vi "MainSimulator_edit.vi"(6 "L2":dbl=130.0, 7 "L1":dbl=100.0, 8 "origin":cluster{"X":dbl, "Y":dbl}={"X"=200.0, "Y"=250.0}, 9 "a":dbl=20.0, 10 "beta 2":dbl(slide)=43.24022346368716 scale=-180.0..180.0, 11 "beta 1":dbl(slide)=43.24022346368716 scale=-180.0..180.0) -> (1 "3D Picture":refnum<vi>(3d-picture), 3 "Canvas":picture)   [LabVIEW 2020]
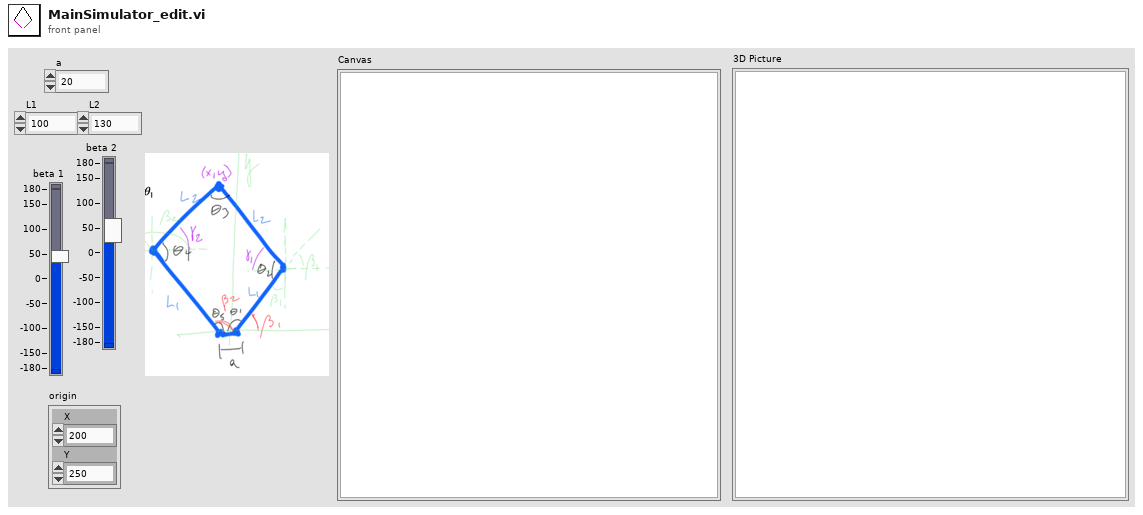
[diagram p1: front panel]
types:
  T1 = cluster{"Color":u32, "Length":dbl, "Base position":cluster{"X":dbl, "Y":dbl}, "Joint Angle":dbl}
  T2 = cluster{"Color":u32, "Length":dbl, "Base position":cluster{"X":dbl, "Y":dbl}, "Joint Angle":dbl}[]
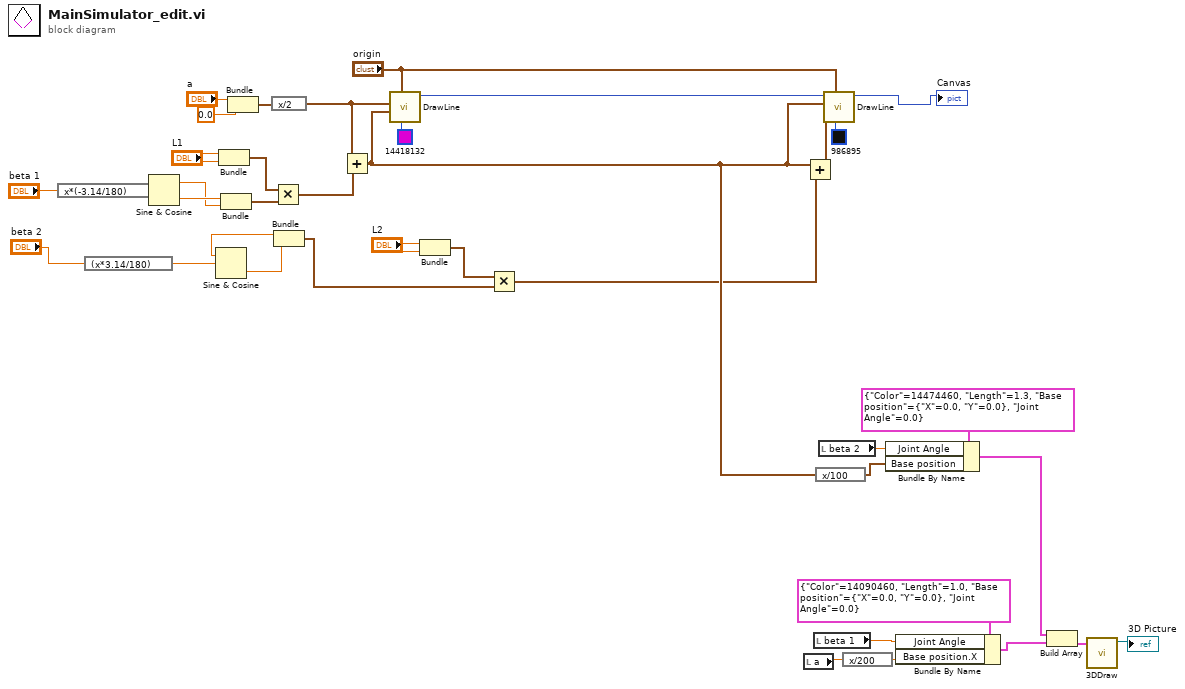
[diagram p0: block diagram]
diagram:
  n1 = expression code="x*(-3.14/180)"("beta 1") -> (w27:dbl)
  n2 = expression code="(x*3.14/180)"("beta 2") -> (w9:dbl)
  n3 = Sine & Cosine(0:w27) -> (1:w32:dbl, 2:w33:dbl)
  n4 = Sine & Cosine(0:w9) -> (1:w7:dbl, 2:w6:dbl)
  n5 = Bundle("L1"="L1", "L1"="L1") -> (w28:cluster{"L1":dbl, "L1":dbl})  [unwired: 1 in]
  n6 = Bundle(w33, w32) -> (w31:cluster{dbl, dbl})  [unwired: 1 in]
  n7 = Bundle("a"="a", 0.0) -> (w35:cluster{"a":dbl, dbl})  [unwired: 1 in]
  n8 = expression code="x/2"(w35) -> (w25:cluster{"a":dbl, dbl})
  n9 = Multiply(x=w28, y=w31) -> (x*y=w30:cluster{dbl, dbl})
  n10 = Bundle(w7, w6) -> (w5:cluster{dbl, dbl})  [unwired: 1 in]
  n11 = Add(x=w25, y=w30) -> (x+y=w14:cluster{dbl, dbl})
  n12 = call "DrawLine.vi"("color(black)"=u32 14418132, "offset"="origin", "move"=w14, "start"=w25) -> ("picture out"=w1:picture)  [unwired: 7 in]
  n13 = Bundle("L2"="L2", "L2"="L2") -> (w26:cluster{"L2":dbl, "L2":dbl})  [unwired: 1 in]
  n14 = Multiply(x=w26, y=w5) -> (x*y=w4:cluster{dbl, dbl})
  n15 = local read "a"() -> (w19:dbl)
  n16 = Add(x=w14, y=w4) -> (x+y=w22:cluster{dbl, dbl})
  n17 = local read "beta 1"() -> (w20:dbl)
  n18 = expression code="x/100"(w14) -> (w13:cluster{dbl, dbl})
  n19 = local read "beta 2"() -> (w10:dbl)
  n20 = call "DrawLine.vi"("color(black)"=u32 986895, "offset"="origin", "move"=w22, "start"=w14, "picture in"=w1) -> ("picture out"=→"Canvas":picture)  [unwired: 6 in]
  n21 = expression code="x/200"(w19) -> (w18:dbl)
  n22 = Bundle By Name(cluster=T1 {"Color"=14474460, "Length"=1.3, "Base position"={"X"=0.0, "Y"=0.0}, "Joint Angle"=0.0} ("Arm"), "Joint Angle"=w10, "Base position"=w13) -> (w12:T1)
  n23 = Bundle By Name(cluster=T1 {"Color"=14090460, "Length"=1.0, "Base position"={"X"=0.0, "Y"=0.0}, "Joint Angle"=0.0} ("Arm"), "Joint Angle"=w20, "Base position.X"=w18) -> (w11:T1)
  n24 = Build Array(w12, w11) -> (w16:T2)
  n25 = call "3DDraw.vi"("Beta/gamma"=w16) -> ("3D Picture"=→"3D Picture":refnum<vi>)  [unwired: 10 in]
